vi "relativepath.vi"() -> ()   [LabVIEW 2018]
panel:
  out "another file":path
  out "same file different diagram":path
  out "current VI's path":path
  out "Current VI's folder":path
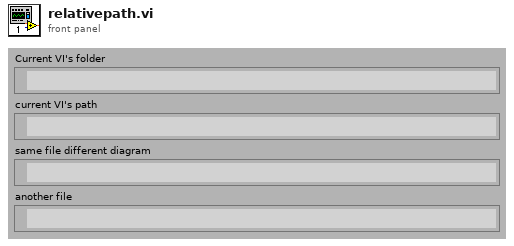
[diagram p1: front panel]
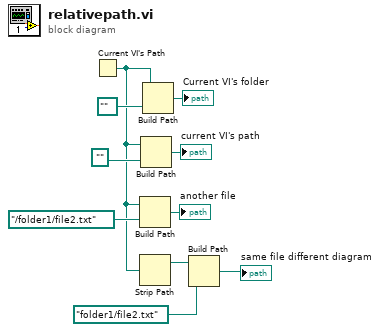
[diagram p0: block diagram]
diagram:
  n1 = Current VI's Path() -> (path=w5:path)
  n2 = Build Path(base path=w5, name or relative path=path "../folder1/file2.txt") -> (appended path=→"another file":path)
  n3 = Strip Path(path=w5) -> (stripped path=w4:path)  [unwired: 1 out]
  n4 = Build Path(base path=w5, name or relative path=path "") -> (appended path=→"current VI's path":path)
  n5 = Build Path(base path=w5, name or relative path=path "..") -> (appended path=→"Current VI's folder":path)
  n6 = Build Path(base path=w4, name or relative path=path "folder1/file2.txt") -> (appended path=→"same file different diagram":path)
